vi "change tag select data type.vi"(7 "data type":T1, 8 "error in":errorcluster, 10 "tag select name":string, 11 "tag select  module configuration in":refnum<class "current tag file io module configuration.lvclass">) -> (0 "error out":errorcluster, 2 "changed channels":refnum<class "TBM channel.lvclass">[](array[class]), 3 "tag select module configuration out":refnum<class "current tag file io module configuration.lvclass">)   [LabVIEW 2013, in "current tag file io module configuration.lvclass"]
uses:
  current tag file io module configuration.lvclass
  <vilib>/NI/Tag Bus/tag/Data Type.ctl
  <vilib>/NI/Tag Bus Module Framework/channel/TBM channel.lvclass
  <vilib>/NI/Tag Bus/tag/tag descriptor.lvclass/tag descriptor.ctl
  current tag file io module configuration.lvclass/current tag file io module configuration.ctl
  <vilib>/NI/Tag Bus/tag/tag descriptor.lvclass
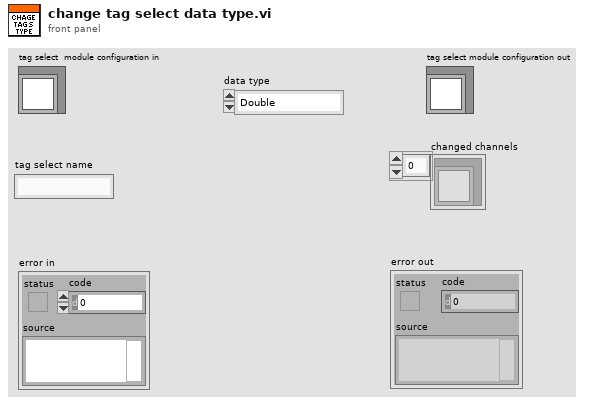
[diagram p1: front panel]
types:
  T1 = typedef "tag bus.lvlib/tag descriptor.lvclass/Data Type.ctl" = enum16{"Double", "Single", "I64", "I32", "I16", "I8", "U64", "U32", "U16", "U8", "Boolean", "String", "Array of Double", "Array of Single", "Array of I64", "Array of I32", "Array of I16", "Array of I8", "Array of U64", "Array of U32", "Array of U16", "Array of U8", "Array of Boolean", "Array of String"}
  T2 = typedef "current tag file io module configuration.lvclass/tag select configuration.ctl" = cluster{"tag select name":string, "data type":T1, "channel":refnum<class "TBM channel.lvclass">}
  T3 = typedef "tag select module configuration.lvclass/tag select configuration.ctl" = cluster{"tag select name":string, "data type":T1, "channel":refnum<class "TBM channel.lvclass">}
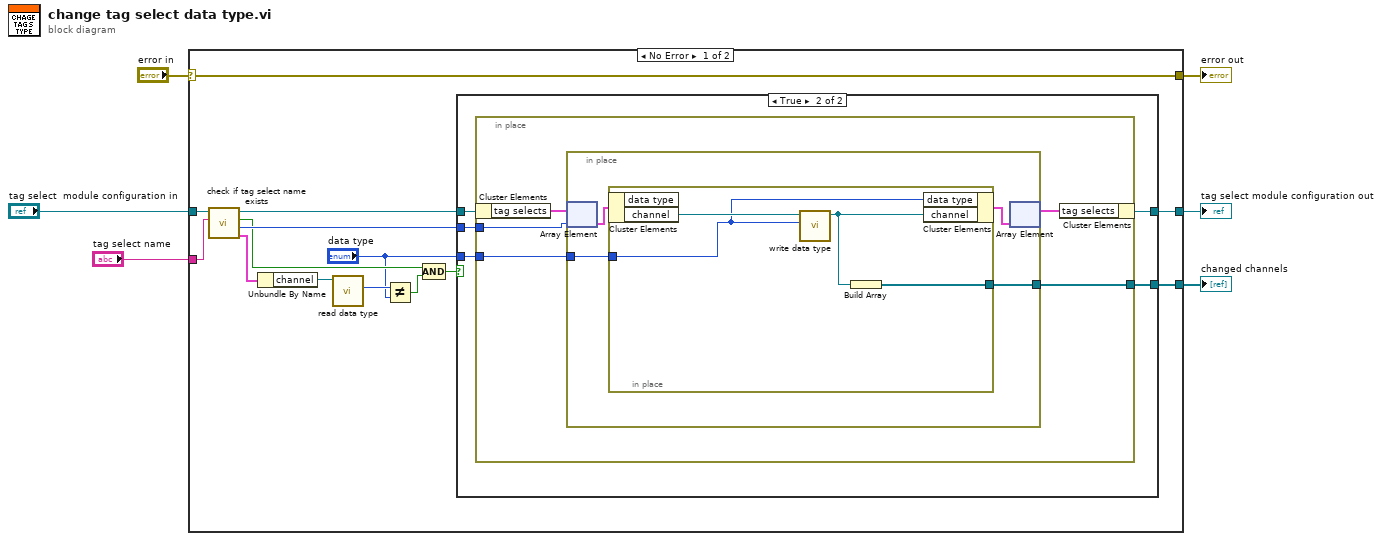
[diagram p0: block diagram]
diagram:
  n1 = case shown="No Error" "error in" {
    selector: "error in" -> [w7 w41]
    tunnel: "tag select  module configuration in" -> [w20 w40]
    tunnel: "tag select name" -> [w19 _]
    tunnel: [w10 _] -> w4
    tunnel: [w9 w40] -> w3
    tunnel: [w7 w41] -> w1
    frame No Error {
      n2 = call "check if tag select name exists.vi"("name to locate"=w19, "tag select module configuration in"=w20) -> ("tag select config"=w16:T2, "index"=w17:i32, "found?"=w13:bool, "tag select module configuration out"=w18:refnum<class "current tag file io module configuration.lvclass">)  [unwired: 6 in]
      n3 = Unbundle By Name(w16) -> ("channel"=w15:refnum<class "TBM channel.lvclass">)
      n4 = call <vilib>:"read data type.vi"("system tag in"=w15) -> ("data type"=w14:T1)  [unwired: 8 in, 2 out]
      n5 = Not Equal?(x=w14, y="data type") -> (x != y?=w12:bool)
      n6 = Compound Arithmetic op=AND(w13, w12) -> (w11:bool)
      n7 = case shown="True" w11 {
        tunnel: w18 -> [w21 w26]
        tunnel: [w21 w25] -> w9
        tunnel: w17 -> [_ w24]
        tunnel: [_ w23] -> w10
        tunnel: "data type" -> [_ w22]
        frame False {
        }
        frame True {
          n8 = in-place {
            in-place-border: w24 -> [w29]
            in-place-border: [w28] -> w23
            in-place-border: w22 -> [w27]
            n9 = in-place-cluster #1(w26) -> ("tag selects"=w31:T3[])
            n10 = in-place {
              in-place-border: [w33] -> w28
              in-place-border: w27 -> [w32]
              n11 = in-place-array #2(w31, w29) -> (w35:T3)
              n12 = in-place {
                in-place-border: [w39] -> w33
                in-place-border: w32 -> [w36]
                n13 = in-place-cluster #3(w35) -> ("channel"=w38:refnum<class "TBM channel.lvclass">)  [unwired: 1 out]
                n14 = call <vilib>:"write data type.vi"("data type"=w36, "system tag in"=w38) -> ("system tag out"=w37:refnum<class "TBM channel.lvclass">)  [unwired: 8 in, 1 out]
                n15 = Build Array(w37) -> (w39:refnum<class "TBM channel.lvclass">[])
                n16 = in-place-cluster #3("data type"=w36, "channel"=w37) -> (w34:T3)
              }
              n17 = in-place-array #2(w34) -> (w30:T3[])  [unwired: 1 out]
            }
            n18 = in-place-cluster #1("tag selects"=w30) -> (w25:refnum<class "current tag file io module configuration.lvclass">)
          }
        }
      }
    }
    frame Error {
    }
  }
  "error out" <- w1
  "tag select module configuration out" <- w3
  "changed channels" <- w4
